vi "Test Epoch Conversions.vi"(8 "error in":errorcluster) -> (0 "error out":errorcluster)   [LabVIEW 2013]
uses:
  source/epoch.UTC/Epoch.UTC.lvclass
  source/epoch/Epoch.lvclass
  source/epoch.GPS/Epoch.GPS.lvclass
  source/epoch.UNIX/Epoch.UNIX.lvclass
  <vilib>/addons/_JKI Toolkits/Caraya/classes/Assert/Assert True.vi
  source/EpochNotTimestamp.vi
  <vilib>/addons/_JKI Toolkits/Caraya/classes/Test/Test.lvclass
  <vilib>/addons/_JKI Toolkits/Caraya/classes/Assert/Assert.lvclass
  <vilib>/addons/_JKI Toolkits/Caraya/classes/Properties/Properties.lvclass
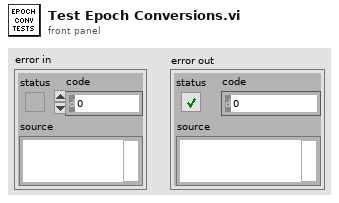
[diagram p1: front panel]
types:
  T1 = cluster{"Label (VI Title)":string, "Epoch Time (s)":i64}
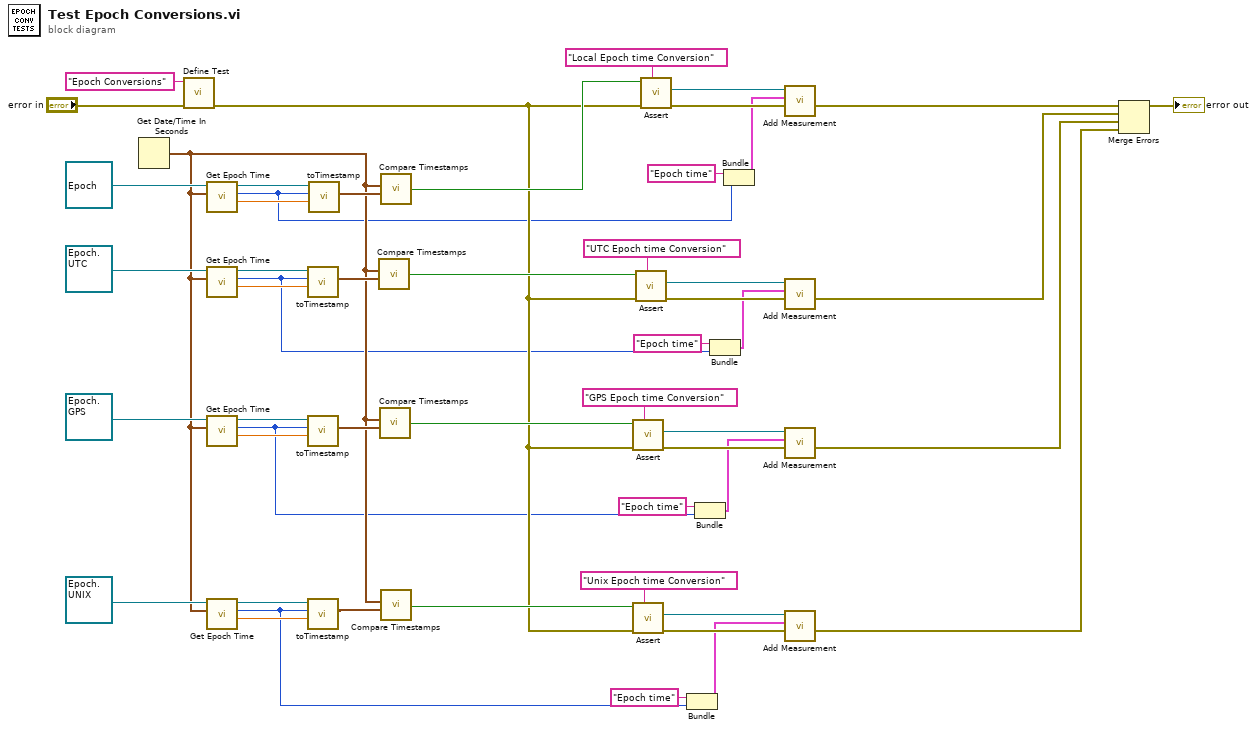
[diagram p0: block diagram]
diagram:
  n1 = Get Date/Time In Seconds() -> (seconds since 1Jan1904=w34:timestamp)
  n2 = call <vilib>:"Define Test.vi"("error in (no error)"="error in", "Label (VI Title)"="Epoch Conversions") -> ("error out"=w14:errorcluster)  [unwired: 8 in, 1 out]
  n3 = call "Get Epoch Time.vi"("Timestamp (now)"=w34, "Epoch (Local)"=refnum<class "Epoch.lvclass"> refnum ("Epoch.lvclass")) -> ("Fractional Second"=w45:dbl, "Epoch Time (s)"=w12:i64, "Epoch out"=w44:refnum<class "Epoch.lvclass">)  [unwired: 7 in]
  n4 = call "Get Epoch Time.vi"("Timestamp (now)"=w34, "Epoch (Local)"=refnum<class "Epoch.UTC.lvclass"> refnum ("Epoch.UTC.lvclass")) -> ("Fractional Second"=w46:dbl, "Epoch Time (s)"=w8:i64, "Epoch out"=w47:refnum<class "Epoch.UTC.lvclass">)  [unwired: 7 in]
  n5 = call "Get Epoch Time.vi"("Timestamp (now)"=w34, "Epoch (Local)"=refnum<class "Epoch.GPS.lvclass"> refnum ("Epoch.GPS.lvclass")) -> ("Fractional Second"=w43:dbl, "Epoch Time (s)"=w3:i64, "Epoch out"=w42:refnum<class "Epoch.GPS.lvclass">)  [unwired: 7 in]
  n6 = call "Get Epoch Time.vi"("Timestamp (now)"=w34, "Epoch (Local)"=refnum<class "Epoch.UNIX.lvclass"> refnum ("Epoch.UNIX.lvclass")) -> ("Fractional Second"=w40:dbl, "Epoch Time (s)"=w4:i64, "Epoch out"=w41:refnum<class "Epoch.UNIX.lvclass">)  [unwired: 7 in]
  n7 = call-dynamic "toTimestamp.vi"("Fractional Second"=w46, "UTC Time (s)"=w8, "Epoch (UTC)"=w47) -> ("Timestamp"=w38:timestamp)  [unwired: 6 in, 2 out]
  n8 = call-dynamic "toTimestamp.vi"("Fractional Second"=w43, "GPS Time (s)"=w3, "Epoch (GPS)"=w42) -> ("Timestamp"=w36:timestamp)  [unwired: 6 in, 2 out]
  n9 = call-dynamic "toTimestamp.vi"("Fractional Second"=w40, "Unix Time (s)"=w4, "Epoch (Unix)"=w41) -> ("Timestamp"=w37:timestamp)  [unwired: 6 in, 2 out]
  n10 = call-dynamic "toTimestamp.vi"("Fractional Second"=w45, "Epoch Time (s)"=w12, "Epoch (Local)"=w44) -> ("Timestamp"=w39:timestamp)  [unwired: 6 in, 2 out]
  n11 = call "Compare Timestamps.vi"("timestamp (1)"=w34, "timestamp (2)"=w38) -> ("Equal?"=w30:bool)  [unwired: 6 in]
  n12 = call "Compare Timestamps.vi"("timestamp (1)"=w34, "timestamp (2)"=w36) -> ("Equal?"=w20:bool)  [unwired: 6 in]
  n13 = call "Compare Timestamps.vi"("timestamp (1)"=w34, "timestamp (2)"=w39) -> ("Equal?"=w33:bool)  [unwired: 6 in]
  n14 = call "Compare Timestamps.vi"("timestamp (1)"=w34, "timestamp (2)"=w37) -> ("Equal?"=w15:bool)  [unwired: 6 in]
  n15 = call-poly <vilib>:"Assert.vi"("Label"="GPS Epoch time Conversion" ("Label (VI Title)"), "error in (no error)"=w14, "True?"=w20) -> ("error out"=w22:errorcluster, "Properties"=w21:refnum<class "Properties.Assert.lvclass">)  [unwired: 7 in]
  n16 = call-poly <vilib>:"Assert.vi"("Label"="Unix Epoch time Conversion" ("Label (VI Title)"), "error in (no error)"=w14, "True?"=w15) -> ("error out"=w17:errorcluster, "Properties"=w18:refnum<class "Properties.Assert.lvclass">)  [unwired: 7 in]
  n17 = call-poly <vilib>:"Assert.vi"("Label"="UTC Epoch time Conversion" ("Label (VI Title)"), "error in (no error)"=w14, "True?"=w30) -> ("error out"=w24:errorcluster, "Properties"=w25:refnum<class "Properties.Assert.lvclass">)  [unwired: 7 in]
  n18 = call-poly <vilib>:"Assert.vi"("Label"="Local Epoch time Conversion" ("Label (VI Title)"), "error in (no error)"=w14, "True?"=w33) -> ("error out"=w27:errorcluster, "Properties"=w28:refnum<class "Properties.Assert.lvclass">)  [unwired: 7 in]
  n19 = Bundle("Label (VI Title)"="Epoch time", "Epoch Time (s)"=w4) -> (w1:T1)  [unwired: 1 in]
  n20 = Bundle("Label (VI Title)"="Epoch time", "Epoch Time (s)"=w3) -> (w2:T1)  [unwired: 1 in]
  n21 = Bundle("Label (VI Title)"="Epoch time", "Epoch Time (s)"=w8) -> (w7:T1)  [unwired: 1 in]
  n22 = Bundle("Label (VI Title)"="Epoch time", "Epoch Time (s)"=w12) -> (w10:T1)  [unwired: 1 in]
  n23 = call <vilib>:"Add Measurement.vi"("error in (no error)"=w27, "entry"=w10, "Properties"=w28) -> ("error out"=w26:errorcluster)  [unwired: 7 in, 1 out]
  n24 = call <vilib>:"Add Measurement.vi"("error in (no error)"=w24, "entry"=w7, "Properties"=w25) -> ("error out"=w23:errorcluster)  [unwired: 7 in, 1 out]
  n25 = call <vilib>:"Add Measurement.vi"("error in (no error)"=w22, "entry"=w2, "Properties"=w21) -> ("error out"=w19:errorcluster)  [unwired: 7 in, 1 out]
  n26 = call <vilib>:"Add Measurement.vi"("error in (no error)"=w17, "entry"=w1, "Properties"=w18) -> ("error out"=w13:errorcluster)  [unwired: 7 in, 1 out]
  n27 = Merge Errors(w26, w23, w19, w13) -> (→"error out":errorcluster)
